vi "PH_O2_Watch.constructor.vi"(0 "name":string, 2 "data in":string, 5 "error in(no error)":errorcluster) -> (14 "i ref out":refnum<vi>, 16 "data out":string, 19 "error out":errorcluster)   [LabVIEW 2014, in "PH_O2_Watch.lvlib"]
doc: "This class is forseen read out the value of an oxid sensor. \n\nThis class is part of the PHELIX device layer.\n\nauthor: Stefan Götte, GSI\n\nLicense Agreement for this software:\n\nCopyright (C)\nGesellschaft für Schwerionenforschung, GSI\nPlanckstr. 1\n64291 Darmstadt\nGermany\n\nContact: D.Beck@gsi.de \n\nThis program is free software; you can redistribute it and/or modify it under the terms of the \nGNU General Public License as published by the Free Software Foundation; either version 2 of \nthe license, or (at your option) any later version.\n\nThis program is distributed in the hope that it will be useful, but WITHOUT ANY WARRANTY; \nwithout even the implied warranty of MERCHANTABILITY or FITNESS FOR A PARTICULAR PURPOSE. See the GNU General License for more details (http://www.gnu.org).\n\nGesellschaft für Schwerionenforschung, GSI\nPlanckstr. 1, 64291 Darmstadt, Germany\nFor all questions and ideas contact: M.Richter@gsi.de, H.Brand@gsi.de or D.Beck@gsi.de.\nLast update: 16-JUN-2004"
uses:
  PH_O2_Watch.lvlib
  PH_O2_Watch.i attribute.ctl
  PH_Basics/PH_StatusHandler/PH_StatusHandler.Status.ctl
  PH_Basics/PH_PSDBWriter/PH_PSDBWriter.lvlib
  PH_Basics/PH_Class/PH_Class.lvlib
  PH_Basics/PH_Common/PH_Common.lvlib
  PH_Basics/PH_StatusHandler/PH_StatusHandler.lvlib
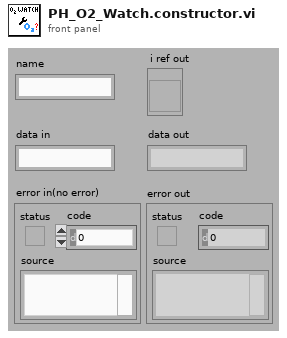
[diagram p1: front panel]
types:
  T1 = typedef "PH_O2_Watch.lvlib/PH_O2_Watch.i attribute.ctl" = cluster{"GUI Refs":cluster{"PreAlert":refnum<vi>, "Alert":refnum<vi>, "Failure":refnum<vi>, "Concentration":refnum<vi>, "Delete":refnum<vi>, "Limit":refnum<vi>}, "State PreAlert":T2, "State Alert":T2, "State Failure":T2, "Concentration":dbl, "Limit":dbl}
  T2 = typedef "PH_StatusHandler.lvlib/PH_StatusHandler.Status.ctl" = i16
  T3 = enum16{"SetAttribute", "GetAttribute", "CreateAttribute", "DestroyAttribute", "DestroyAllAtributes"}
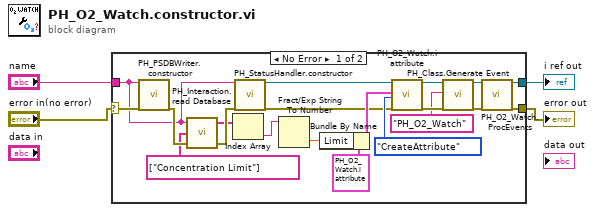
[diagram p0: block diagram]
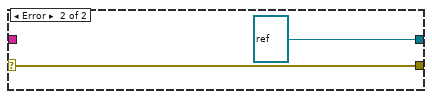
[diagram p2: hidden frame]
diagram:
  n1 = case shown="No Error" "error in(no error)" {
    selector: "error in(no error)" -> [w24 w26]
    tunnel: "name" -> [w5 _]
    tunnel: [w12 w26] -> w3
    tunnel: [w15 refnum<vi> refnum ("i ref out")] -> w2
    frame No Error {
      n2 = call "PH_PSDBWriter.constructor.vi"("name"=w5, "error in"=w24) -> ("error out"=w23:errorcluster)  [unwired: 15 in, 2 out]
      n3 = call "PH_Interaction.read Database.vi"("error in (no error)"=w23, "Strings to search for"=string[] ["Concentration Limit"], "DB Entry to read"=w5) -> ("error out"=w10:errorcluster, "Values"=w8:string[])  [unwired: 1 in]
      n4 = Index Array(array=w8) -> (element=w9:string)  [unwired: 1 in]
      n5 = call "PH_StatusHandler.constructor.vi"("name"=w5, "error in(no error)"=w10) -> ("i ref out"=w18:refnum<vi>, "error out"=w19:errorcluster)  [unwired: 15 in, 1 out]
      n6 = Fract/Exp String To Number(string=w9) -> (number=w7:dbl)  [unwired: 3 in, 1 out]
      n7 = Bundle By Name(cluster=T1 {"GUI Refs"={"PreAlert"=refnum, "Alert"=refnum, "Failure"=refnum, "Concentration"=refnum, "Delete"=refnum, "Limit"=refnum}, "State PreAlert"=0, "State Alert"=0, "State Failure"=0, "Concentration"=0.0, "Limit"=0.0} ("CLASS.i attribute"), "Limit"=w7) -> (w20:T1)
      n8 = call "PH_O2_Watch.i attribute.vi"("VI Refnum"=w18, "CLASS.i attribute"=w20, "Action"=T3."CreateAttribute", "error in (no error)"=w19) -> ("VI Refnum out"=w17:refnum<vi>, "error out"=w14:errorcluster)  [unwired: 13 in, 1 out]
      n9 = call "PH_Class.Generate Event.vi"("i ref in"=w17, "Class"="PH_O2_Watch", "error in (no error)"=w14) -> ("i ref out"=w16:refnum<vi>, "error out"=w13:errorcluster)  [unwired: 15 in]
      n10 = call "PH_O2_Watch.ProcEvents.vi"("i ref in"=w16, "error in (no error)"=w13) -> ("i ref out"=w15:refnum<vi>, "error out"=w12:errorcluster)  [unwired: 16 in]
    }
    frame Error {
    }
  }
  "i ref out" <- w2
  "error out" <- w3
